vi "PS FPGA Filter Read Coefficients.vi"(11 "offset":u16) -> (2 "a coeffs":fxp<+/-,22,4>[](array[numeric]), 3 "b coeffs":fxp<+/-,22,4>[](array[numeric]))   [LabVIEW 2011]
uses:
  <vilib>/rvi/Memory/Memory_Emulation/niFpgaMemoryEmulationValidateCache.vi
  <vilib>/rvi/DataTransferAndStorage/Container/Common/niFpgaContainerGetUniqueNameForEmu.vi
  <vilib>/rvi/Memory/Memory_Emulation/nirvimemoryEmulationManagerCache_InsertValue.vi
  <vilib>/Utility/error.llb/Clear Errors.vi
  <vilib>/rvi/Memory/Memory_Emulation/nirvimemoryEmulationManagerCache_GetValue.vi
  <vilib>/rvi/DataTransferAndStorage/Container/XNode/niFpgaContainer.xnode
  <vilib>/rvi/Memory/Memory_Emulation/nirvimemoryEmulation.vi
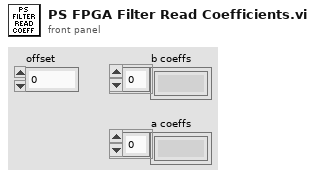
[diagram p1: front panel]
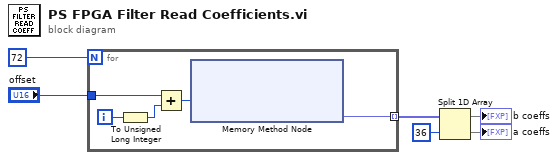
[diagram p0: block diagram]
diagram:
  n1 = for {
    N: 72 ("Number of\nCoefficients\nper Channel") -> [_]
    tunnel: [w8] -> w3 mode=indexing
    tunnel: "offset" -> [w7]
    i -> [w11]
    n2 = To Unsigned Long Integer(number=w11) -> (unsigned 32bit integer=w10:u32)
    n3 = Add(x=w7, y=w10) -> (x+y=w9:u32)
    n4 = xnode ("Memory Method Node")("Address"=w9) -> ("Data"=w8:fxp<+/-,22,4>)  [unwired: 1 in, 1 out]
  }
  n5 = Split 1D Array(array=w3, index=36) -> (first subarray=→"b coeffs":fxp<+/-,22,4>[], second subarray=→"a coeffs":fxp<+/-,22,4>[])
